vi "Main.vi"() -> ()   [LabVIEW 2016]
doc: "Use this template to build a simple state machine design pattern. Each state executes code and determines which state to transition to."
uses:
  Mediciones/controls/Estados.ctl
  <instrlib>/Stanford Research 830/Stanford Research 830.lvlib
  <instrlib>/Stanford Research 830/Public/Data/Read (All Parameters).vi
  Mediciones/controls/process.ctl
  <vilib>/silver_ctls/ArrayMatrixCluster/Real Matrix NI_Silver.ctl
  Mediciones/controls/Parameters.ctl
  Mediciones/controls/Lambda.ctl
  Mediciones/controls/LockIn.ctl
  Mediciones/controls/lamp.ctl
  Mediciones/controls/monochromator.ctl
  Mediciones/controls/powermeter.ctl
panel:
  in  "Exit":bool
  in  "Components":T1(tab)
  in  "Normalize":bool
  out "Graphics":cluster{dbl, dbl}(graph)
  out "Process":T2 {"Samples" format="%#_4g"; "Stabilizing" scale=0.0..100.0; "Lambda" scale=0.0..100.0; "Sample" scale=0.0..100.0}
  in  "Measure":bool
  in  "Save":bool
  in  "Parameters":T4={"Lambda"={"Init"=350.0, "Final"=700.0, "dx"=5.0}, "Power"=400.0, "Frequency"=0.0, "Stabilizing"=10.0, "Samples"=100.0, "File"=path ""}
  in  "Monochromator":T6={"Port"="", "Connected"=FALSE, "Lambda"=350.0, "Shutter"=FALSE, "Lamp-model"="", "Open"=FALSE, "Save"=FALSE, "Grid"={"Number"=1, "Min"=0.0, "Max"=0.0}, "GPIB"=""} {"Grid"."Number" items=["1"=1, "2"=2]}
  in  "Lamp":T7={"Port"="", "Power"=200, "Is Conected?"=FALSE, "ON"=FALSE, "Open"=FALSE, "Save"=FALSE, "Model"=""} {"Power" min=200 max=1000 step=1 scale=200.0..1000.0}
  in  "Lock-In-Amplifier":T8={"Port"="", "Is connected?"=FALSE, "Sensivity Ovld"=FALSE, "lockin-open"=FALSE, "lockin-save"=FALSE, "Reference"={"Source "=0, "Frequency"=1000.0}, "Channel Display"={"Channel 1"=1, "Channel 2"=1}, "Sensivity"={"Dynamic Reserve"=0, "Sensitivity"=25, "Time Constant"=11, "Low Pass Filter"=2}, "Display"={"Channel One"=0.0, "Channel Two"=0.0, "Reference"=0.0}, "Parameter Values"={"X-Value"=0.0, "Y-Value"=0.0, "R-Value"=0.0, "Theta-Value"=0.0, "Aux In 1 Value"=0.0, "Aux In 2 Value"=0.0, "Aux In 3 Value"=0.0, "Aux In 4 Value"=0.0, "Reference Frequency"=0.0, "Channel 1 Display"=0.0, "Channel 2 Display"=0.0}} {"Display"."Reference" format="%#_6p"; "Display"."Channel Two" format="%#_6p"; "Display"."Channel One" format="%#_6p"; "Sensivity"."Low Pass Filter" items=["6 dB/oct", "12 dB/oct", "18 db/oct", "24 dB/oct"]; "Sensivity"."Time Constant" items=["10 us", "30 us", "100 us", "300 us", "1 ms", "3 ms", "10 ms", "30 ms", "100 ms", "300 ms", "1 s", "3 s", "10 s", "30 s", "100 s", "300 s", "1 ks", "3 ks", "10 ks", "30 ks"]; "Sensivity"."Sensitivity" items=["Auto Gain"=-1, "2 nV/fA"=0, "5 nV/fA"=1, "10 nV/fA"=2, "20 nV/fA"=3, "50 nV/fA"=4, "100 nV/fA"=5, "200 nV/fA"=6, "500 nV/fA"=7, "1 uV/pA"=8, "2 uV/pA"=9, "5 uV/pA"=10, "10 uV/pA"=11, "20 uV/pA"=12, "50 uV/pA"=13, "100 uV/pA"=14, "200 uV/pA"=15, "500 uV/pA"=16, "1 mV/nA"=17, "2 mV/nA"=18, "5 mV/nA"=19, "10 mV/nA"=20, "20 mV/nA"=21, "50 mV/nA"=22, "100 mV/nA"=23, "200 mV/nA"=24, "500 mV/mA"=25, "1 V/uA"=26]; "Sensivity"."Dynamic Reserve" items=["Auto Reserve"=-1, "High Reserve"=0, "Normal"=1, "Low Noise"=2]; "Channel Display"."Channel 2" items=["Y", "Theta", "Y Noise", "Aux In 3", "Aux In 4"]; "Channel Display"."Channel 1" items=["X", "R", "X Noise", "Aux In 1", "Aux In 2"]; "Reference"."Source" items=["External", "Internal"]}
  in  "Power Meter":T9 {"Dev. Std." format="%#_5p"; "Lambda" format="%#_6p"; "Power" format="%#_5p"}
  out "Graphic Real":T10(graph)
  in  "Save Power":bool
  in  "DataPower":dbl[][](array[numeric])
  in  "Power Data":dbl[][](array[numeric])
  in  "File Power":path
  out "Power Spectra":cluster{dbl, dbl}(graph)
  in  "Spectra":bool
  # "Hz"
  # "s"
  # "W"
  # "nm"
  # "nm"
  # "nm"
  # "Measure"
  # "INSTITUTO POLITECNICO NACIONAL\nCENTRO DE INVESTIGACIONES EN CIENCIA APLICADA Y TECNOLOGÍA AVANZADA\n\nPHOTOTHERMAL  ESPECTROMETER"
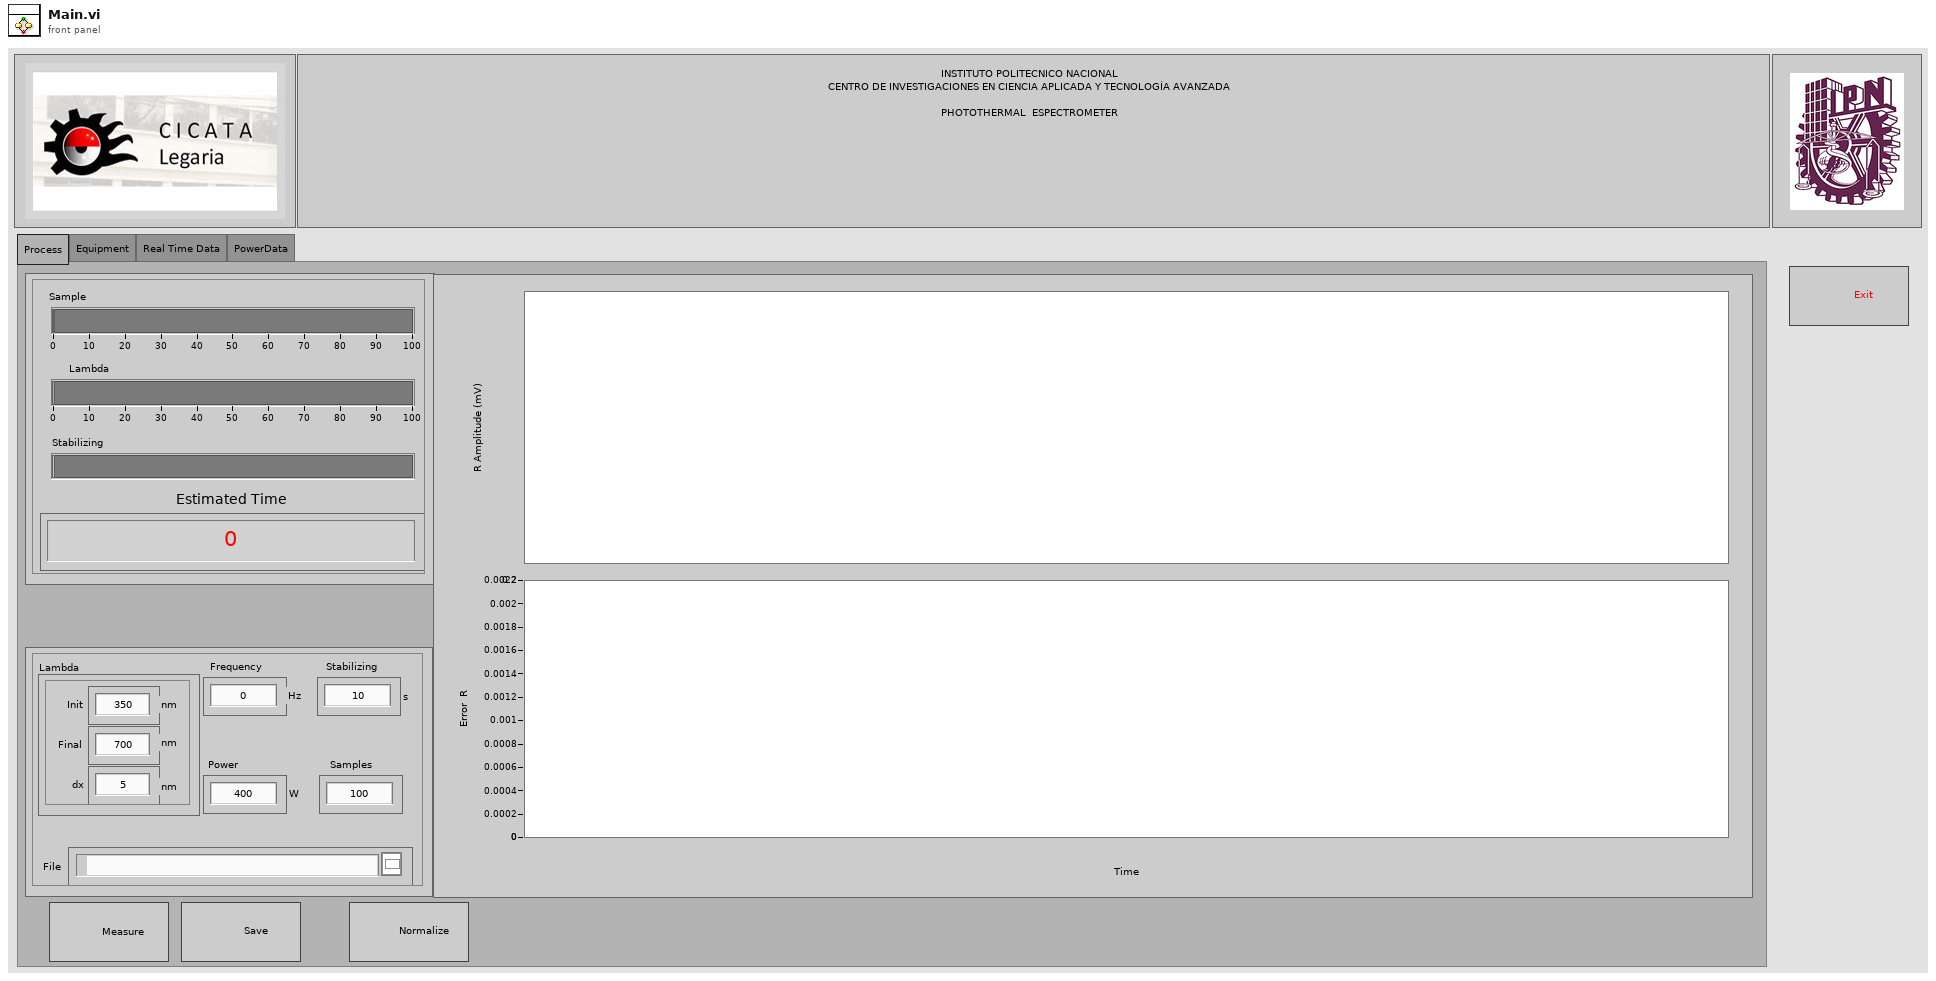
[diagram p1: front panel]
types:
  T1 = enum32{"Process", "Equipment", "Real Time Data", "PowerData"}
  T2 = typedef "process.ctl" = cluster{"Sample":u16, "Lambda":u16, "Stabilizing":u16, "Status":u8, "Estimated Time":dbl, "Samples":T3, "Data":T3, "Lambda-Index":dbl, "Graph":bool}
  T3 = typedef "Real Matrix NI_Silver.ctl" = dbl[][]
  T4 = typedef "Parameters.ctl" = cluster{"Lambda":T5, "Power":dbl, "Frequency":dbl, "Stabilizing":dbl, "Samples":dbl, "File":path}
  T5 = typedef "Lambda.ctl" = cluster{"Init":dbl, "Final":dbl, "dx":dbl}
  T6 = typedef "monochromator.ctl" = cluster{"Port":refnum<visa-resource-name>, "Connected":bool, "Lambda":dbl, "Shutter":bool, "Lamp-model":string, "Open":bool, "Save":bool, "Grid":cluster{"Number":u8, "Min":dbl, "Max":dbl}, "GPIB":string}
  T7 = typedef "lamp.ctl" = cluster{"Port":refnum<visa-resource-name>, "Power":u16, "Is Conected?":bool, "ON":bool, "Open":bool, "Save":bool, "Model":string}
  T8 = typedef "LockIn.ctl" = cluster{"Port":refnum<visa-resource-name>, "Is connected?":bool, "Sensivity Ovld":bool, "lockin-open":bool, "lockin-save":bool, "Reference":cluster{"Source ":u16, "Frequency":dbl}, "Channel Display":cluster{"Channel 1":u16, "Channel 2":u16}, "Sensivity":cluster{"Dynamic Reserve":i16, "Sensitivity":i16, "Time Constant":u16, "Low Pass Filter":u16}, "Display":cluster{"Channel One":dbl, "Channel Two":dbl, "Reference":dbl}, "Parameter Values":cluster{"X-Value":dbl, "Y-Value":dbl, "R-Value":dbl, "Theta-Value":dbl, "Aux In 1 Value":dbl, "Aux In 2 Value":dbl, "Aux In 3 Value":dbl, "Aux In 4 Value":dbl, "Reference Frequency":dbl, "Channel 1 Display":dbl, "Channel 2 Display":dbl}}
  T9 = typedef "powermeter.ctl" = cluster{"Start":bool, "Serial ":string, "Model":string, "Sensor":string, "Power":dbl, "Density":bool, "Lambda":dbl, "Open":bool, "Save":bool, "reference":refnum<k7>, "hDevice":i32, "Dev. Std.":dbl, "Channel":i16}
  T10 = cluster{"X-Value":dbl, "Y-Value":dbl, "R-Value":dbl, "Theta-Value":dbl}
  T11 = typedef "Estados.ctl" = enum16{"Inicializar", "Evento", "Salir"}
  T12 = cluster{"X-Value":dbl, "Y-Value":dbl, "R-Value":dbl, "Theta-Value":dbl}[]
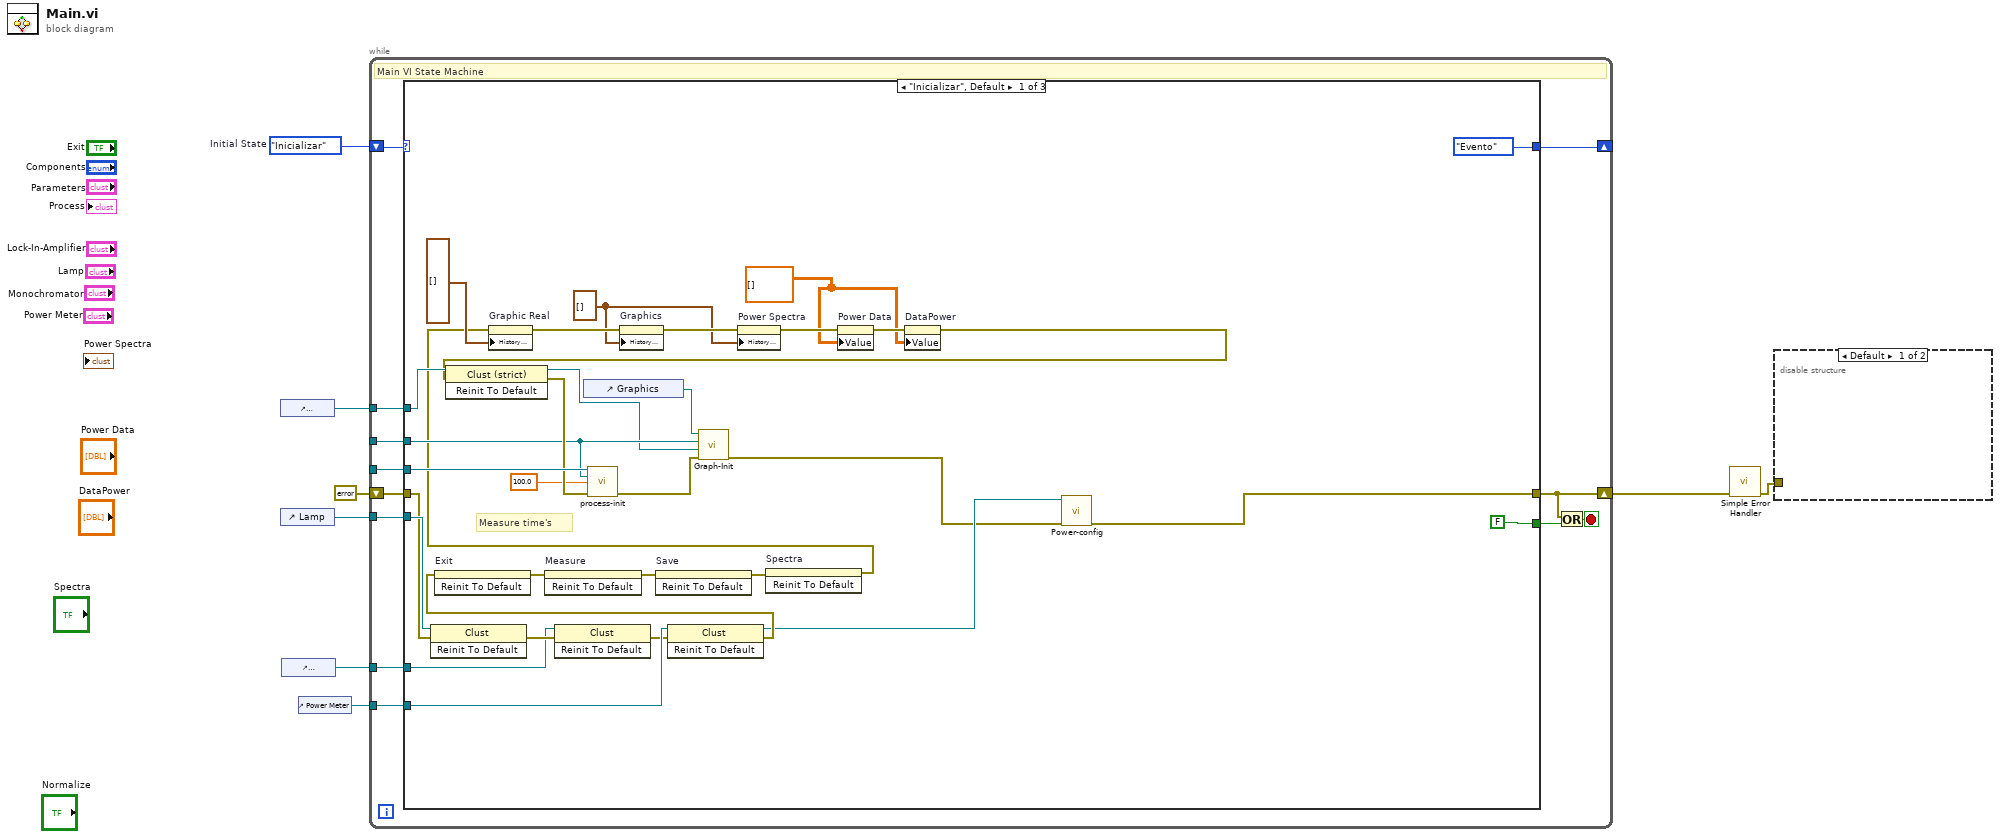
[diagram p0: block diagram]
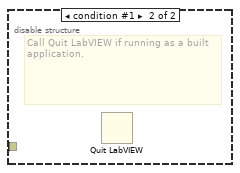
[diagram p2: hidden frame]
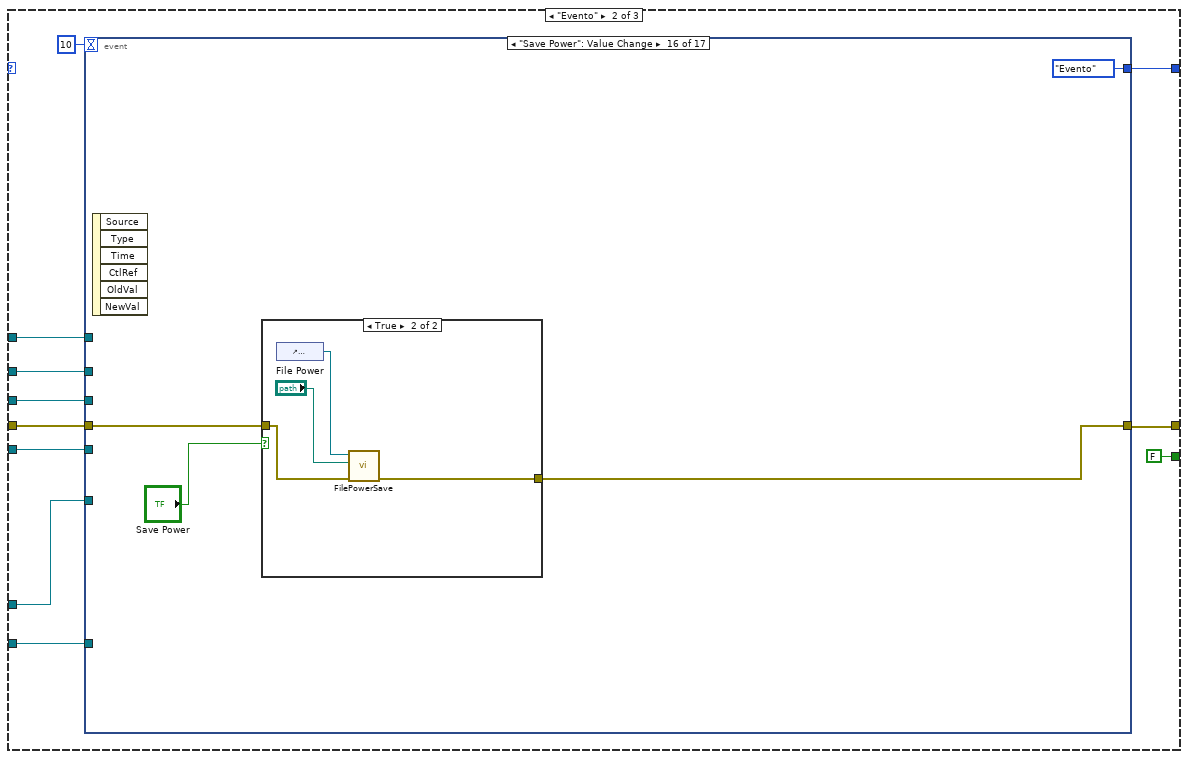
[diagram p3: hidden frame]
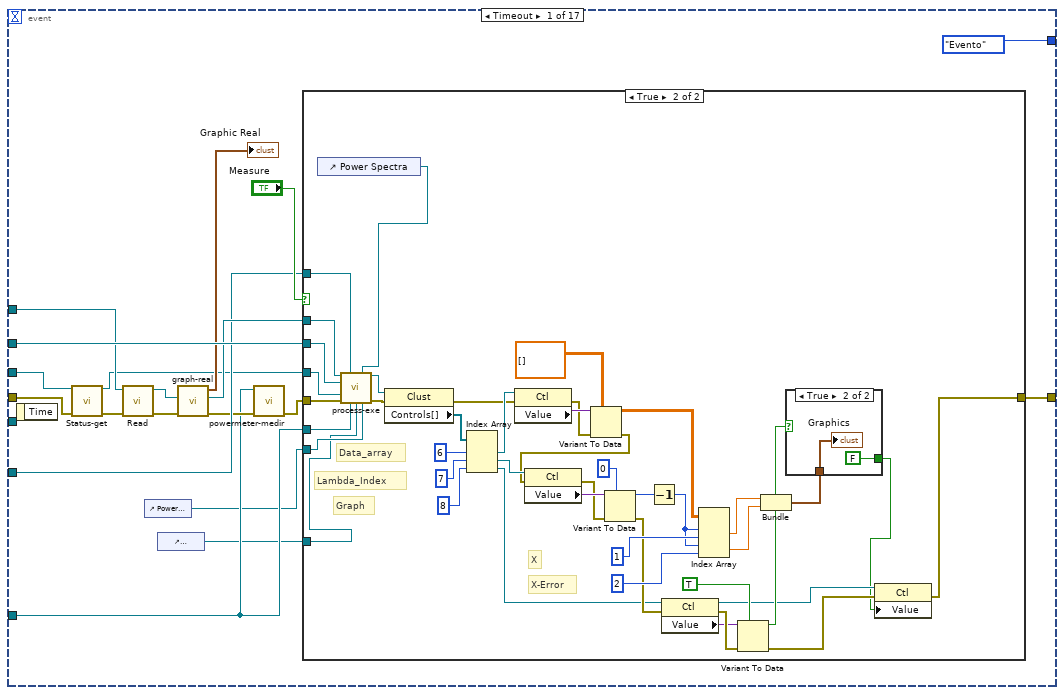
[diagram p4: hidden frame]
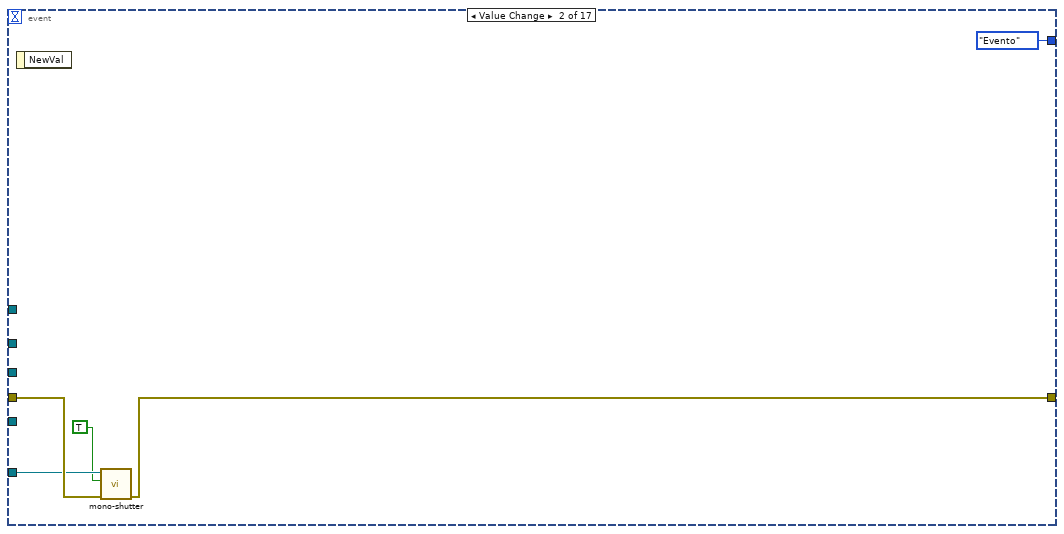
[diagram p7: hidden frame]
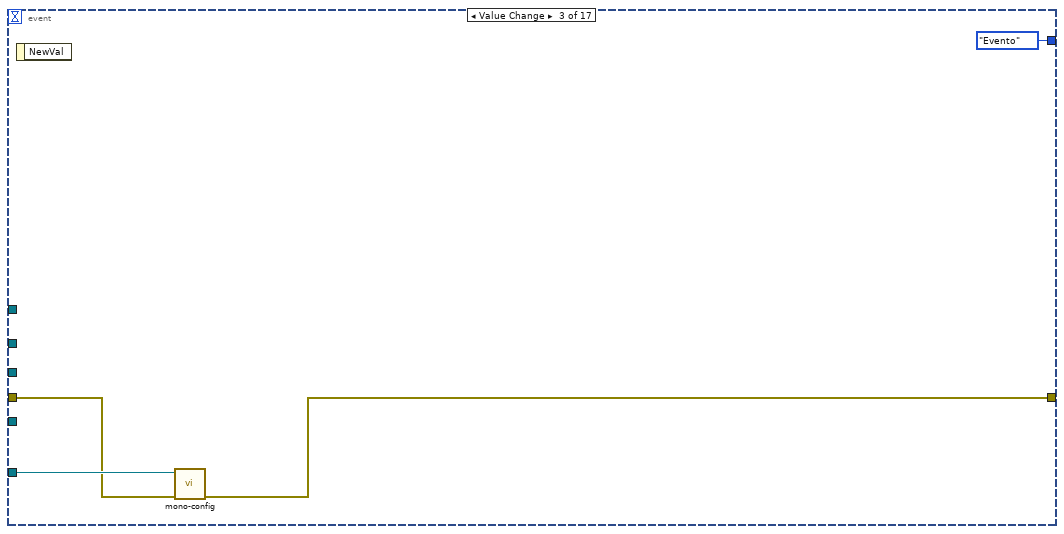
[diagram p8: hidden frame]
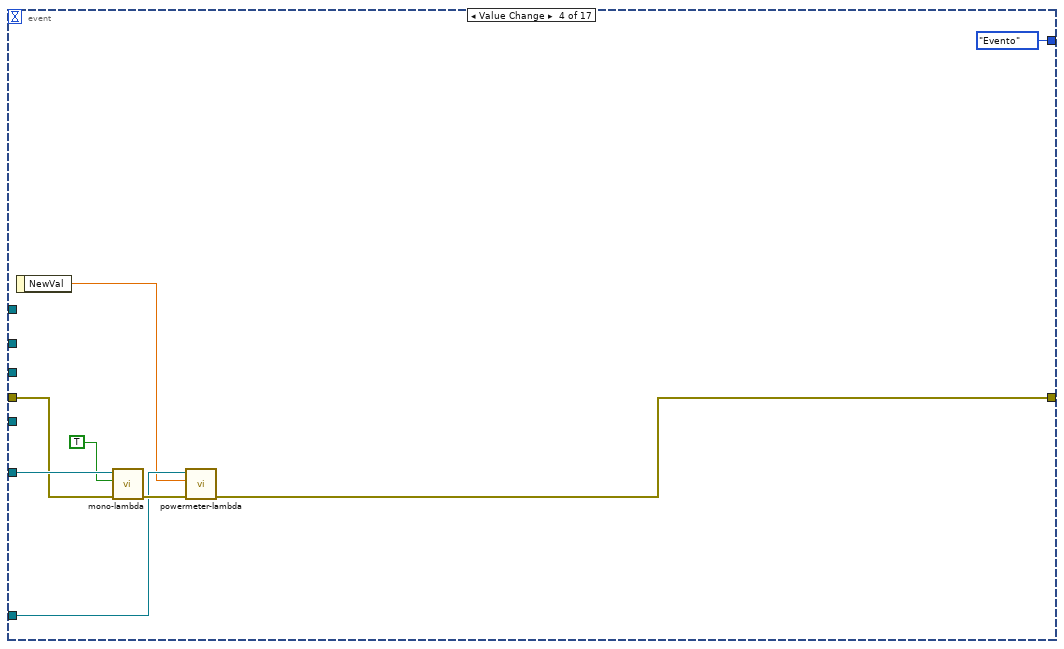
[diagram p9: hidden frame]
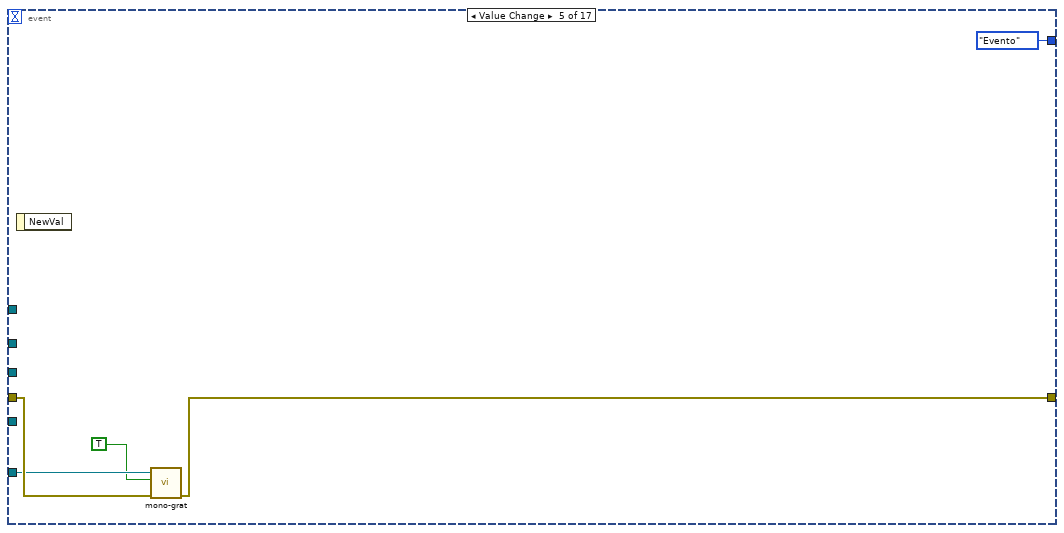
[diagram p10: hidden frame]
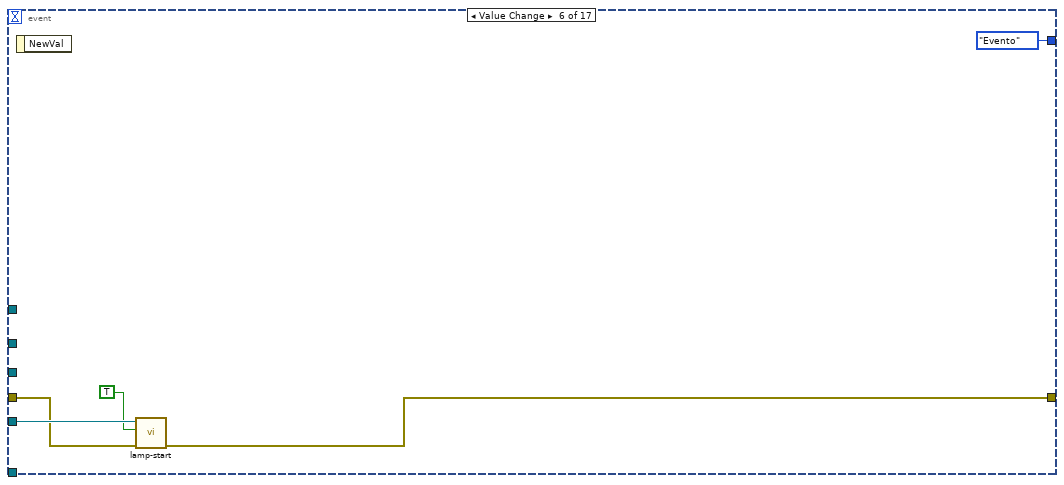
[diagram p11: hidden frame]
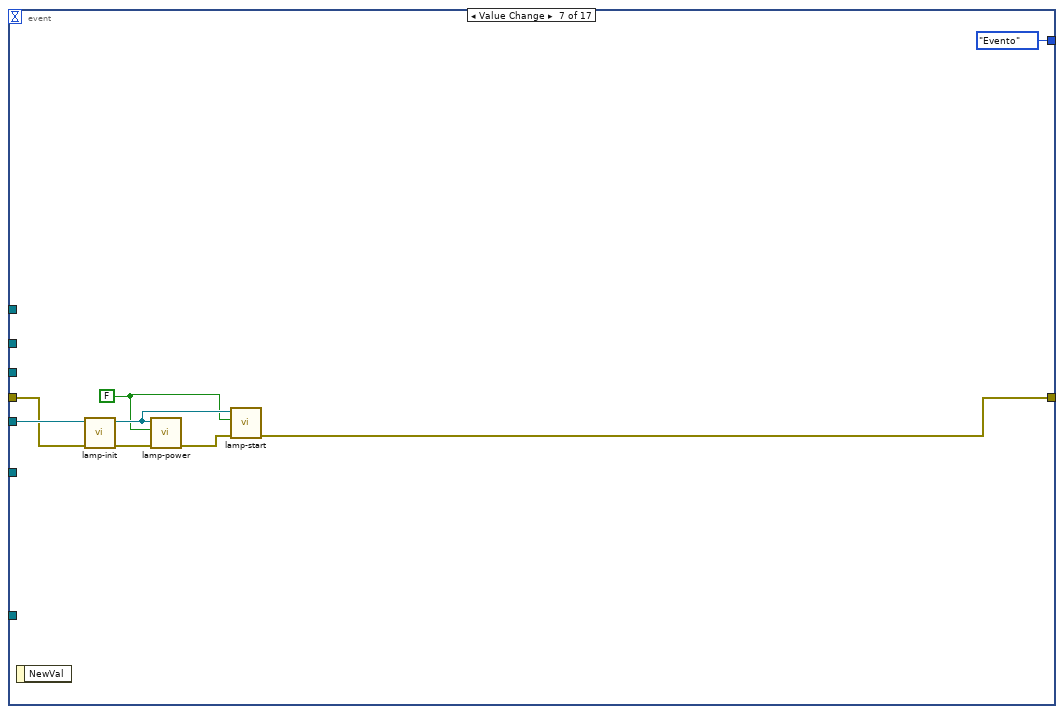
[diagram p12: hidden frame]
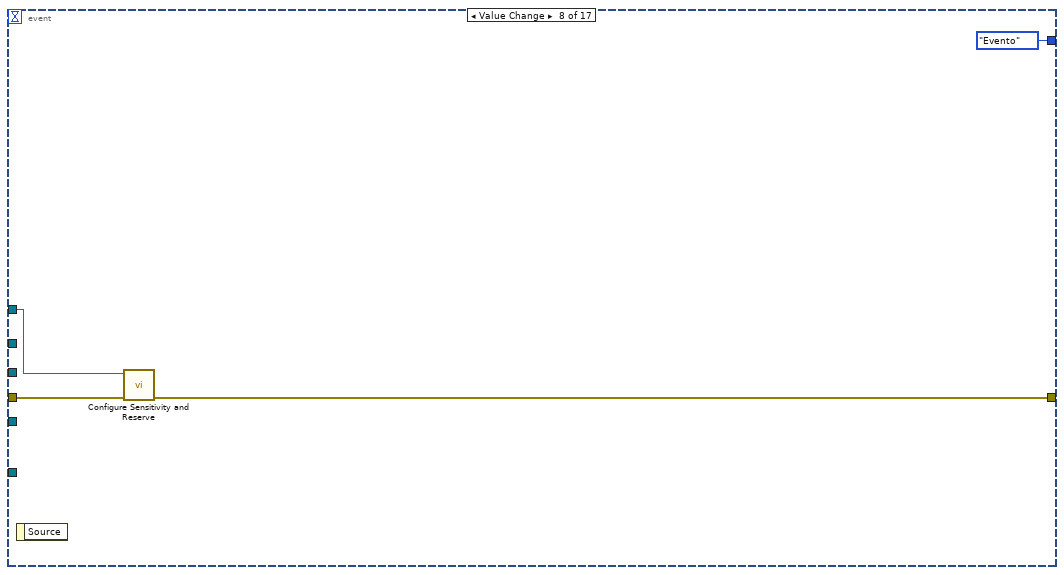
[diagram p13: hidden frame]
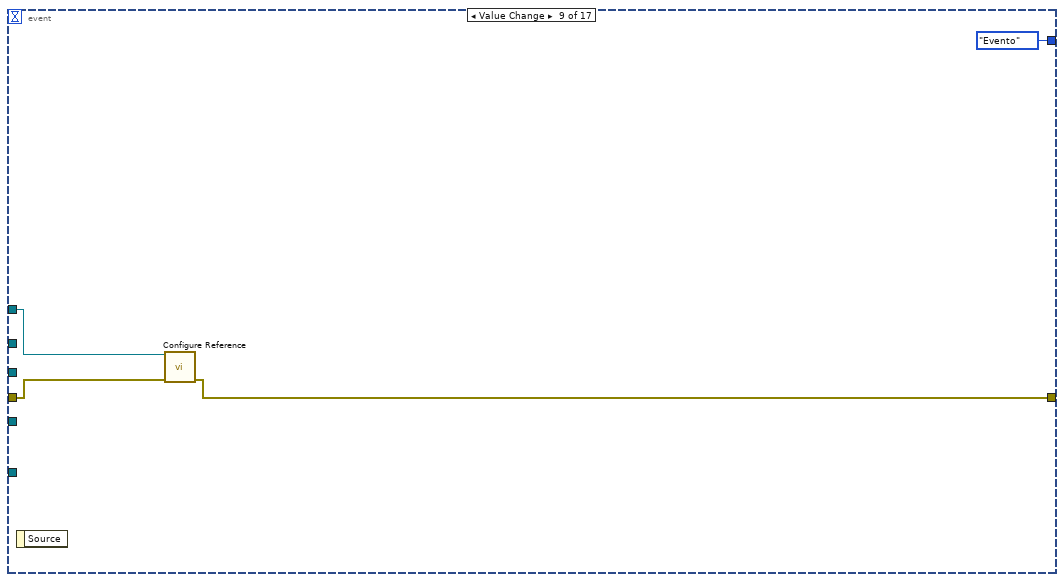
[diagram p14: hidden frame]
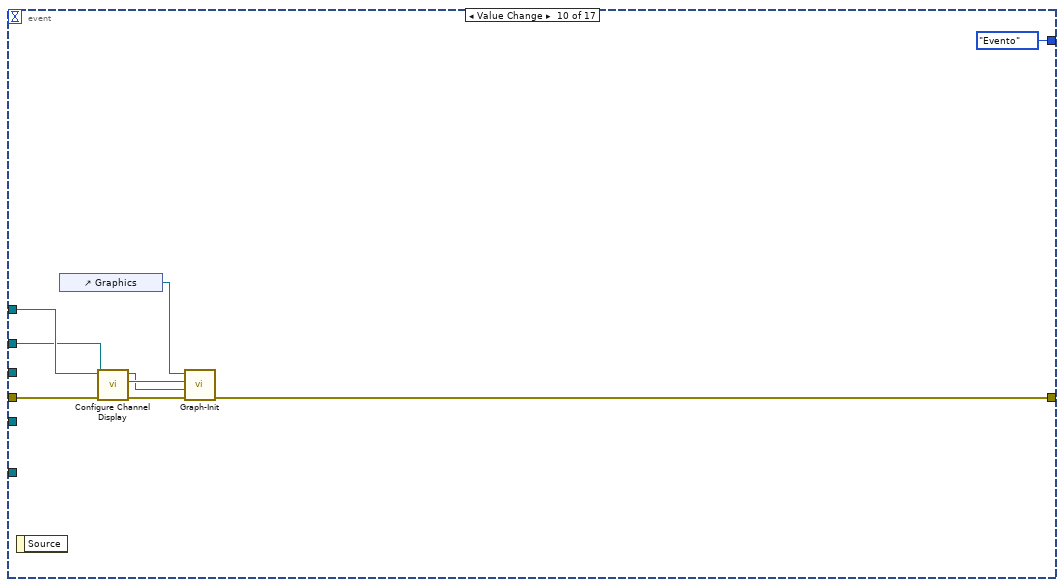
[diagram p15: hidden frame]
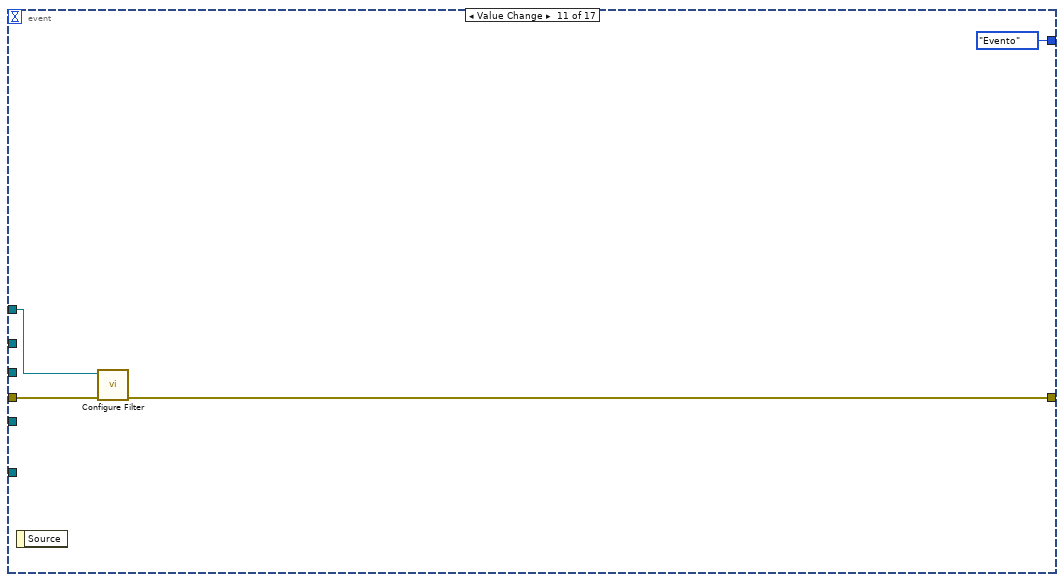
[diagram p16: hidden frame]
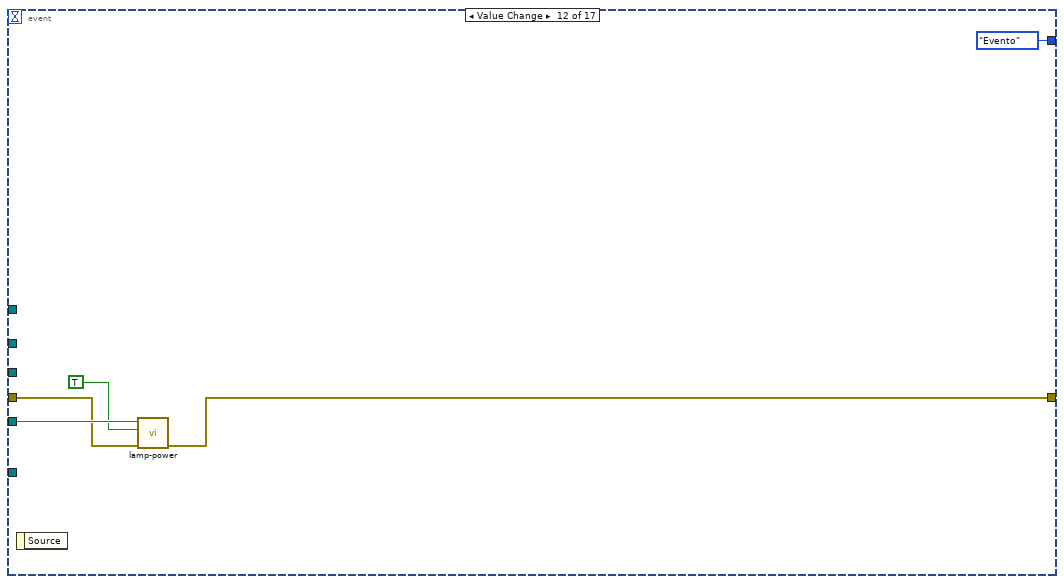
[diagram p17: hidden frame]
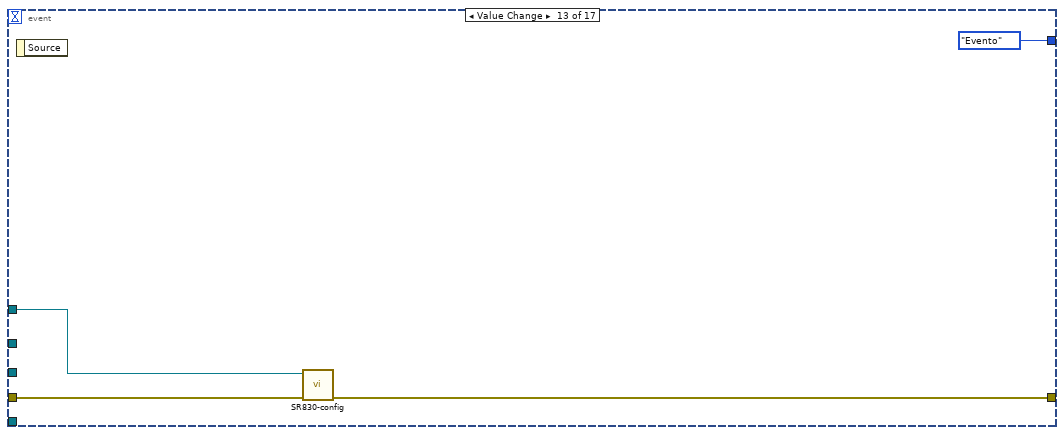
[diagram p18: hidden frame]
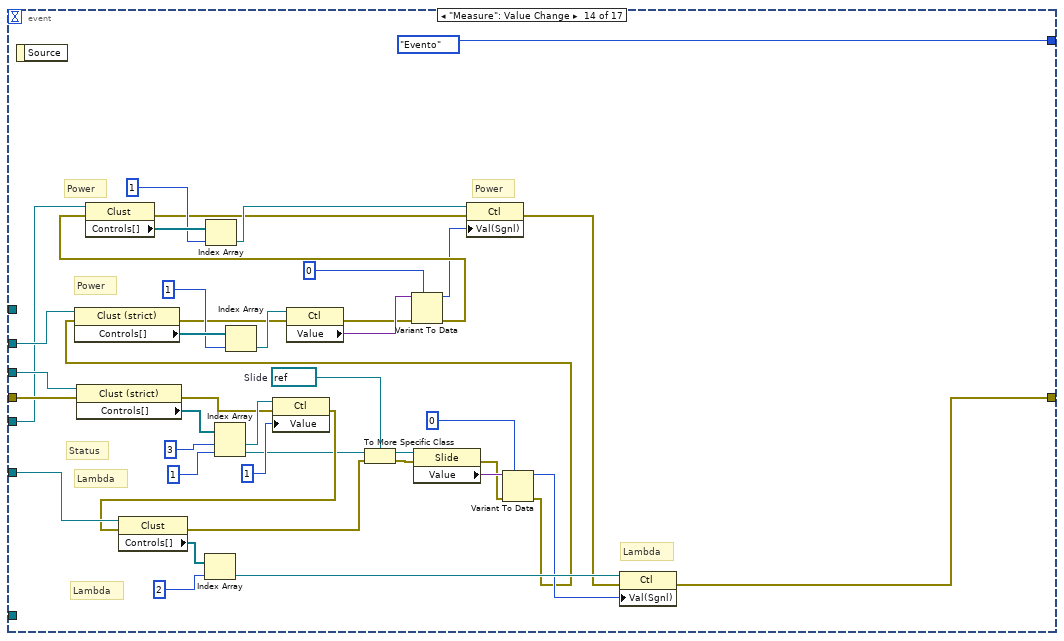
[diagram p19: hidden frame]
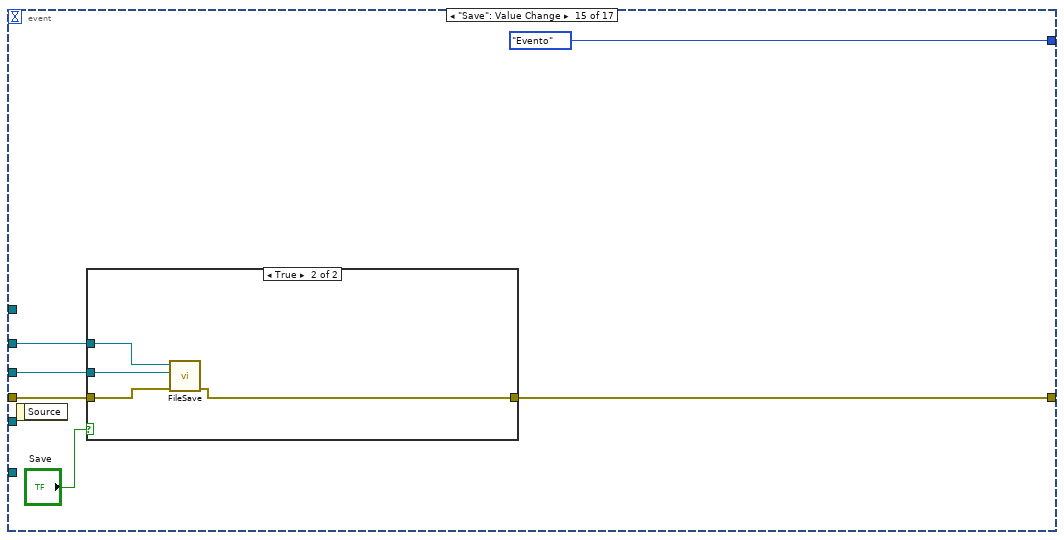
[diagram p20: hidden frame]
diagram:
  w10 = Estados."Inicializar"  # Initial State
  n1 = control-ref of="Lock-In-Amplifier"() -> (w5:refnum<vi>)
  n2 = control-ref of="Lamp"() -> (w2:refnum<vi>)
  n3 = control-ref of="Monochromator"() -> (w3:refnum<vi>)
  n4 = control-ref of="Power Meter"() -> (w4:refnum<vi>)
  n5 = while {
    shift-right: [w17] -> _
    shift-left: w10 -> [w21]
    shift-right: [w20] -> w8
    shift-left: errorcluster {"status"=FALSE, "code"=0, "source"=""} ("error constant") -> [w19]
    tunnel: w5 -> [w14]
    tunnel: [w15] -> w6
    tunnel: [w16] -> w1
    tunnel: w2 -> [w13]
    tunnel: w3 -> [w12]
    tunnel: w4 -> [w11]
    stop <- w22 stop-if-true
    # "Main VI State Machine"
    n6 = case shown="\"Inicializar\", Default" w21 {
      tunnel: [w29 w61 w262] -> w20
      tunnel: w19 -> [w41 w62 w262]
      tunnel: [FALSE FALSE TRUE] -> w18
      tunnel: [Estados."Evento" ("Initial State") w60 Estados."Salir" ("Initial State")] -> w17
      tunnel: w16 -> [w52 w64 _]
      tunnel: w15 -> [w44 w63 _]
      tunnel: w14 -> [w51 w59 _]
      tunnel: w13 -> [w42 w58 _]
      tunnel: w12 -> [w39 w57 _]
      tunnel: w11 -> [w34 w56 _]
      frame "Inicializar", Default {
        w23 = dbl[][] []
        w27 = cluster{dbl, dbl}[] [] ("History Data")
        # "Measure time's"
        n7 = invoke class="Clust" method="Reinit To Default"(reference=w42, error in=w41) -> (error out=w40:errorcluster)  [unwired: 1 in, 2 out]
        n8 = invoke class="Clust" method="Reinit To Default"(reference=w39, error in=w40) -> (error out=w33:errorcluster)  [unwired: 1 in, 2 out]
        n9 = control-ref of="Graphics"() -> (w45:refnum<vi>)
        n10 = invoke class="Clust" method="Reinit To Default"(reference=w34, error in=w33) -> (reference out=w31:refnum<vi>, error out=w32:errorcluster)  [unwired: 1 in, 1 out]
        n11 = invoke on="Exit" class="Bool" method="Reinit To Default"(error in=w32) -> (error out=w49:errorcluster)  [unwired: 2 in, 2 out]
        n12 = invoke on="Measure" class="Bool (strict)" method="Reinit To Default"(error in=w49) -> (error out=w48:errorcluster)  [unwired: 2 in, 2 out]
        n13 = invoke on="Save" class="Bool" method="Reinit To Default"(error in=w48) -> (error out=w36:errorcluster)  [unwired: 2 in, 2 out]
        n14 = invoke on="Spectra" class="Bool (strict)" method="Reinit To Default"(error in=w36) -> (error out=w35:errorcluster)  [unwired: 2 in, 2 out]
        n15 = property on="Graphic Real" class="WFChart (strict)"(error in=w35, "History Data"=T12 []) -> (error out=w47:errorcluster)  [unwired: 1 in, 1 out]
        n16 = property on="Graphics" class="WFChart (strict)"(error in=w47, "History Data"=w27) -> (error out=w28:errorcluster)  [unwired: 1 in, 1 out]
        n17 = property on="Power Spectra" class="WFChart (strict)"(error in=w28, "History Data"=w27) -> (error out=w26:errorcluster)  [unwired: 1 in, 1 out]
        n18 = property on="Power Data" class="Arr (strict)"(error in=w26, "Value"=w23) -> (error out=w25:errorcluster)  [unwired: 1 in, 1 out]
        n19 = property on="DataPower" class="Arr (strict)"(error in=w25, "Value"=w23) -> (error out=w24:errorcluster)  [unwired: 1 in, 1 out]
        n20 = invoke class="Clust (strict)" method="Reinit To Default"(reference=w51, error in=w24) -> (reference out=w37:refnum<vi>, error out=w50:errorcluster)  [unwired: 1 in, 1 out]
        n21 = call "process-init.vi"("Process In"=w52, "Parameter"=w44, "Time"=100.0, "Error In"=w50) -> ("Error Out"=w46:errorcluster)  [unwired: 9 in, 2 out]
        n22 = call "Graph-Init.vi"("error in (no error)"=w46, "SR830 in"=w37, "Parameters"=w44, "WaveformChart in"=w45) -> ("error out"=w30:errorcluster)  [unwired: 7 in]
        n23 = call "Power-config.vi"("error in (no error)"=w30, "powermeter in"=w31) -> ("error out"=w29:errorcluster)  [unwired: 9 in]
      }
      frame "Evento" {
        n24 = event shown="[15] \"Save Power\": Value Change" {
          selector: _ -> [_ _ _ _ _ _ _ _ _ _ _ _ _ _ _ _ _]
          dyn-events: _ -> [_ _ _ _ _ _ _ _ _ _ _ _ _ _ _ _ _]
          timeout: 10 -> [_ _ _ _ _ _ _ _ _ _ _ _ _ _ _ _ _]
          tunnel: w64 -> [w76 _ _ _ _ _ _ _ _ _ _ _ _ w235 w239 _ _]
          tunnel: w63 -> [w82 _ _ _ _ _ _ _ _ w178 _ _ _ w211 w240 _ _]
          tunnel: [w74 w132 w136 w142 w149 w154 w158 w167 w171 w175 w183 w187 w193 w212 w236 w247 w257] -> w61
          tunnel: w62 -> [w80 w135 w137 w146 w152 w155 w164 w168 w172 w180 w185 w188 w194 w229 w238 w248 w258]
          tunnel: [Estados."Evento" ("Initial State") Estados."Evento" ("Initial State") Estados."Evento" ("Initial State") Estados."Evento" ("Initial State") Estados."Evento" ("Initial State") Estados."Evento" ("Initial State") Estados."Evento" ("Initial State") Estados."Evento" ("Initial State") Estados."Evento" ("Initial State") Estados."Evento" ("Initial State") Estados."Evento" ("Initial State") Estados."Evento" ("Initial State") Estados."Evento" ("Initial State") Estados."Evento" ("Initial State") Estados."Evento" ("Initial State") Estados."Evento" ("Initial State") Estados."Salir" ("Initial State")] -> w60
          tunnel: w59 -> [w77 _ _ _ _ _ _ w169 w173 w181 w184 _ w191 _ _ _ w256]
          tunnel: w58 -> [_ _ _ _ _ w156 w165 _ _ _ _ w189 _ w205 _ _ _]
          tunnel: w57 -> [w72 w134 w138 w147 w151 _ _ _ _ _ _ _ _ w224 _ _ _]
          tunnel: w56 -> [w68 _ _ w141 _ _ _ _ _ _ _ _ _ _ _ _ _]
          event Timeout {
            n25 = event-data() -> ()  [unwired: 1 in, 1 out]
            n26 = call "Status-get.vi"("Process in"=w76) -> ("Process out"=w71:refnum<vi>)  [unwired: 10 in, 4 out]
            n27 = call-poly <instrlib>:"Read.vi"("error in"=w80, "SR830 in"=w77) -> ("error out"=w79:errorcluster, "Sr830 out"=w78:refnum<vi>)  [unwired: 8 in]
            n28 = control-ref of="Power Data"() -> (w67:refnum<vi>)
            n29 = control-ref of="DataPower"() -> (w66:refnum<vi>)
            n30 = call "graph-real.vi"("error in (no error)"=w79, "Sr830 in"=w78) -> ("error out"=w69:errorcluster, "Sr830 out"=w75:refnum<vi>, "Data"=→"Graphic Real":T10)  [unwired: 7 in]
            n31 = call "powermeter-medir.vi"("error in (no error)"=w69, "Powermeter"=w68) -> ("error out"=w70:errorcluster)  [unwired: 9 in]
            n32 = case shown="True" "Measure" {
              tunnel: w71 -> [_ w126]
              tunnel: [w84 w91] -> w74
              tunnel: w82 -> [_ w127]
              tunnel: w75 -> [_ w125]
              tunnel: w70 -> [w84 w124]
              tunnel: w72 -> [_ w89]
              tunnel: w68 -> [_ w88]
              tunnel: w67 -> [_ w86]
              tunnel: w66 -> [_ w85]
              frame False {
              }
              frame True {
                # "Graph"
                # "X-Error"
                # "X"
                # "Lambda_Index"
                # "Data_array"
                n33 = control-ref of="Power Spectra"() -> (w87:refnum<vi>)
                n34 = call "process-exe.vi"("SR830 in"=w125, "Monochromator"=w89, "PowerGraph"=w87, "Parameters"=w127, "Process In"=w126, "error in"=w124, "Powermeter"=w88, "Arr Power"=w85, "Arr Refnum"=w86) -> ("Process out"=w104:refnum<vi>, "error out"=w121:errorcluster)  [unwired: 5 in]
                n35 = property class="Clust"(reference=w104, error in=w121) -> (error out=w115:errorcluster, "Controls[]"=w120:refnum<vi>[])  [unwired: 1 out]
                n36 = Index Array(array=w120, index #1=6 ("index"), index #2=7 ("index"), index #3=8 ("index")) -> (element #1=w116:refnum<vi>, element #2=w111:refnum<vi>, element #3=w101:refnum<vi>)
                n37 = property class="Ctl"(reference=w116, error in=w115) -> (error out=w117:errorcluster, "Value"=w118:variant)  [unwired: 1 out]
                n38 = Variant To Data(error in=w117, type=dbl[][] [], Variant=w118) -> (data=w105:dbl[][], error out=w110:errorcluster)
                n39 = property class="Ctl"(reference=w111, error in=w110) -> (error out=w113:errorcluster, "Value"=w114:variant)  [unwired: 1 out]
                n40 = Variant To Data(error in=w113, type=0, Variant=w114) -> (data=w109:i32, error out=w102:errorcluster)
                n41 = Decrement(x=w109) -> (x-1=w106:i32)
                n42 = property class="Ctl"(reference=w101, error in=w102) -> (reference out=w93:refnum<vi>, error out=w100:errorcluster, "Value"=w99:variant)
                n43 = Index Array(array=w105, index (row) #1=w106, index (col) #1=1 ("disabled index (col)"), index (row) #2=w106, index (col) #2=2 ("disabled index (col)")) -> (element #1=w96:dbl, element #2=w95:dbl)
                n44 = Variant To Data(error in=w100, type=TRUE, Variant=w99) -> (data=w97:bool, error out=w92:errorcluster)
                n45 = Bundle(w96, w95) -> (w94:cluster{dbl, dbl})  [unwired: 1 in]
                n46 = case shown="True" w97 {
                  selector: w97 -> [w128 _]
                  tunnel: w94 -> [_ w130]
                  tunnel: [w128 FALSE] -> w90
                  frame False {
                  }
                  frame True {
                    "Graphics" <- w130
                  }
                }
                n47 = property class="Ctl"(reference=w93, error in=w92, "Value"=w90) -> (error out=w91:errorcluster)  [unwired: 1 out]
              }
            }
          }
          event Value Change {
            n48 = event-data() -> ()  [unwired: 1 in, 1 out]
            n49 = call "mono-shutter.vi"("error in (no error)"=w135, "Set"=TRUE, "Monochromator"=w134) -> ("error out"=w132:errorcluster)  [unwired: 8 in]
          }
          event Value Change {
            n50 = event-data() -> ()  [unwired: 1 in, 1 out]
            n51 = call "mono-config.vi"("error in (no error)"=w137, "Monochromator"=w138) -> ("error out"=w136:errorcluster)  [unwired: 9 in]
          }
          event Value Change {
            n52 = event-data() -> ("NewVal"=w140:dbl)  [unwired: 1 in]
            n53 = call "mono-lambda.vi"("Error In"=w146, "set"=TRUE, "Monochromator"=w147) -> ("Error Out"=w143:errorcluster)  [unwired: 8 in]
            n54 = call "powermeter-lambda.vi"("error in (no error)"=w143, "Lambda"=w140, "PowerMeter"=w141) -> ("error out"=w142:errorcluster)  [unwired: 7 in, 1 out]
          }
          event Value Change {
            n55 = event-data() -> ()  [unwired: 1 in, 1 out]
            n56 = call "mono-grat.vi"("Error In"=w152, "Set"=TRUE, "Mono"=w151) -> ("Error Out"=w149:errorcluster)  [unwired: 8 in]
          }
          event Value Change {
            n57 = event-data() -> ()  [unwired: 1 in, 1 out]
            n58 = call "lamp-start.vi"("error in (no error)"=w155, "Set"=TRUE, "Lamp"=w156) -> ("error out"=w154:errorcluster)  [unwired: 8 in]
          }
          event Value Change {
            w160 = FALSE ("Set")
            n59 = event-data() -> ()  [unwired: 1 in, 1 out]
            n60 = call "lamp-init.vi"("error in (no error)"=w164, "Lamp"=w165) -> ("error out"=w162:errorcluster, "Lamp Out"=w161:refnum<vi>)  [unwired: 8 in]
            n61 = call "lamp-power.vi"("error in (no error)"=w162, "Set"=w160, "Lamp"=w161) -> ("error out"=w159:errorcluster)  [unwired: 8 in]
            n62 = call "lamp-start.vi"("error in (no error)"=w159, "Set"=w160, "Lamp"=w161) -> ("error out"=w158:errorcluster)  [unwired: 8 in]
          }
          event Value Change {
            n63 = event-data() -> ()  [unwired: 1 in, 1 out]
            n64 = call <instrlib>:"Configure Sensitivity and Reserve.vi"("error in"=w168, "SR830 in"=w169) -> ("error out"=w167:errorcluster)  [unwired: 8 in, 1 out]
          }
          event Value Change {
            n65 = event-data() -> ()  [unwired: 1 in, 1 out]
            n66 = call <instrlib>:"Configure Reference.vi"("SR830 in"=w173, "error in (no error)"=w172) -> ("error out"=w171:errorcluster)  [unwired: 12 in, 1 out]
          }
          event Value Change {
            n67 = event-data() -> ()  [unwired: 1 in, 1 out]
            n68 = control-ref of="Graphics"() -> (w177:refnum<vi>)
            n69 = call <instrlib>:"Configure Channel Display.vi"("error in"=w180, "SR830 in"=w181) -> ("error out"=w176:errorcluster, "Sr830 out"=w174:refnum<vi>)  [unwired: 8 in]
            n70 = call "Graph-Init.vi"("error in (no error)"=w176, "SR830 in"=w174, "Parameters"=w178, "WaveformChart in"=w177) -> ("error out"=w175:errorcluster)  [unwired: 7 in]
          }
          event Value Change {
            n71 = event-data() -> ()  [unwired: 1 in, 1 out]
            n72 = call <instrlib>:"Configure Filter.vi"("error in"=w185, "SR830 in"=w184) -> ("error out"=w183:errorcluster)  [unwired: 8 in, 1 out]
          }
          event Value Change {
            n73 = event-data() -> ()  [unwired: 1 in, 1 out]
            n74 = call "lamp-power.vi"("error in (no error)"=w188, "Set"=TRUE, "Lamp"=w189) -> ("error out"=w187:errorcluster)  [unwired: 8 in]
          }
          event Value Change {
            n75 = event-data() -> ()  [unwired: 1 in, 1 out]
            n76 = call "SR830-config.vi"("error in (no error)"=w194, "SR830"=w191) -> ("error out"=w193:errorcluster)  [unwired: 9 in]
          }
          event "Measure": Value Change {
            w220 = refnum<vi> refnum  # Slide
            # "Power"
            # "Power"
            # "Power"
            # "Lambda"
            # "Lambda"
            # "Lambda"
            # "Status"
            n77 = event-data() -> ()  [unwired: 1 in, 1 out]
            n78 = property class="Clust (strict)"(reference=w235, error in=w229) -> (error out=w231:errorcluster, "Controls[]"=w234:refnum<vi>[])  [unwired: 1 out]
            n79 = Index Array(array=w234, index #1=3 ("index"), index #2=1 ("index")) -> (element #1=w232:refnum<vi>, element #2=w221:refnum<vi>)
            n80 = property class="Ctl"(reference=w232, error in=w231, "Value"=1) -> (error out=w223:errorcluster)  [unwired: 1 out]
            n81 = property class="Clust"(reference=w224, error in=w223) -> (error out=w219:errorcluster, "Controls[]"=w227:refnum<vi>[])  [unwired: 1 out]
            n82 = Index Array(array=w227, index=2) -> (element=w225:refnum<vi>)
            n83 = To More Specific Class(target class=w220, reference=w221, error in=w219) -> (specific class reference=w217:refnum<vi>, error out=w218:errorcluster)
            n84 = property class="Slide"(reference=w217, error in=w218) -> (error out=w215:errorcluster, "Value"=w216:variant)  [unwired: 1 out]
            n85 = Variant To Data(error in=w215, type=0, Variant=w216) -> (data=w213:i32, error out=w210:errorcluster)
            n86 = property class="Clust (strict)"(reference=w211, error in=w210) -> (error out=w206:errorcluster, "Controls[]"=w209:refnum<vi>[])  [unwired: 1 out]
            n87 = Index Array(array=w209, index=1) -> (element=w207:refnum<vi>)
            n88 = property class="Ctl"(reference=w207, error in=w206) -> (error out=w203:errorcluster, "Value"=w204:variant)  [unwired: 1 out]
            n89 = Variant To Data(error in=w203, type=0, Variant=w204) -> (data=w196:i32, error out=w201:errorcluster)
            n90 = property class="Clust"(reference=w205, error in=w201) -> (error out=w197:errorcluster, "Controls[]"=w200:refnum<vi>[])  [unwired: 1 out]
            n91 = Index Array(array=w200, index=1) -> (element=w198:refnum<vi>)
            n92 = property class="Ctl"(reference=w198, error in=w197, "Val(Sgnl)"=w196) -> (error out=w195:errorcluster)  [unwired: 1 out]
            n93 = property class="Ctl"(reference=w225, error in=w195, "Val(Sgnl)"=w213) -> (error out=w212:errorcluster)  [unwired: 1 out]
          }
          event "Save": Value Change {
            n94 = event-data() -> ()  [unwired: 1 in, 1 out]
            n95 = case shown="True" "Save" {
              tunnel: w240 -> [_ w246]
              tunnel: w239 -> [_ w245]
              tunnel: w238 -> [w242 w244]
              tunnel: [w242 w243] -> w236
              frame False {
              }
              frame True {
                n96 = call "FileSave.vi"("error in (no error)"=w244, "Process"=w245, "Parameters In"=w246) -> ("error out"=w243:errorcluster)  [unwired: 8 in]
              }
            }
          }
          event "Save Power": Value Change {
            n97 = event-data() -> ()  [unwired: 1 in, 6 out]
            n98 = case shown="True" "Save Power" {
              tunnel: w248 -> [w251 w255]
              tunnel: [w251 w254] -> w247
              frame False {
              }
              frame True {
                n99 = control-ref of="DataPower"() -> (w252:refnum<vi>)
                n100 = call "FilePowerSave.vi"("error in (no error)"=w255, "File Power"="File Power", "Data"=w252) -> ("error out"=w254:errorcluster)  [unwired: 8 in]
              }
            }
          }
          event "Exit": Value Change {
            n101 = event-data() -> ()  [unwired: 1 in, 1 out]
            n102 = call <instrlib>:"Close.vi"("error in"=w258, "SR830 in"=w256) -> ("error out"=w257:errorcluster)  [unwired: 9 in]
          }
        }
      }
      frame "Salir" {
      }
    }
    n103 = Or(x=w20, y=w18) -> (x .or. y?=w22:bool)
  }
  n104 = call <vilib>:"Simple Error Handler.vi"("error in (no error)"=w8) -> ("error out"=w7:errorcluster)  [unwired: 4 in, 4 out]
  n105 = disable-structure shown="Default" {
    disable-tunnel: w7 -> [_ _]
    frame condition #0 (active) {
    }
    frame condition #1 {
      # "Call Quit LabVIEW if running as a built application."
      n106 = Quit LabVIEW() -> ()  [unwired: 1 in]
    }
  }
